vi "Demo Global.vi"() -> ()   [LabVIEW 2019]
doc: "A global variable used by the tutorial to show how channels can negate the need to use a global variable."
panel:
  out "latest value":i32
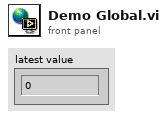
[diagram p1: front panel]
diagram:
